vi "XY Galvo.vi"(0 "Exposure /ms":dbl=10.0 format="%0.2p", 1 "FOV max / V":dbl=10.0 format="%0.2p", 2 "Samples per ms":dbl=10.0 format="%0.2p", 3 "Relax /ms":dbl=10.0 format="%0.2p", 4 "FOV min/ V":dbl=10.0 format="%0.2p") -> (5 "XY Galvo":dbl[](graph))   [LabVIEW 2015]
uses:
  GlobalVariables.vi
  <vilib>/Analysis/NI_AALBase.lvlib
panel:
  out "XY Galvo 2":dbl[](graph)
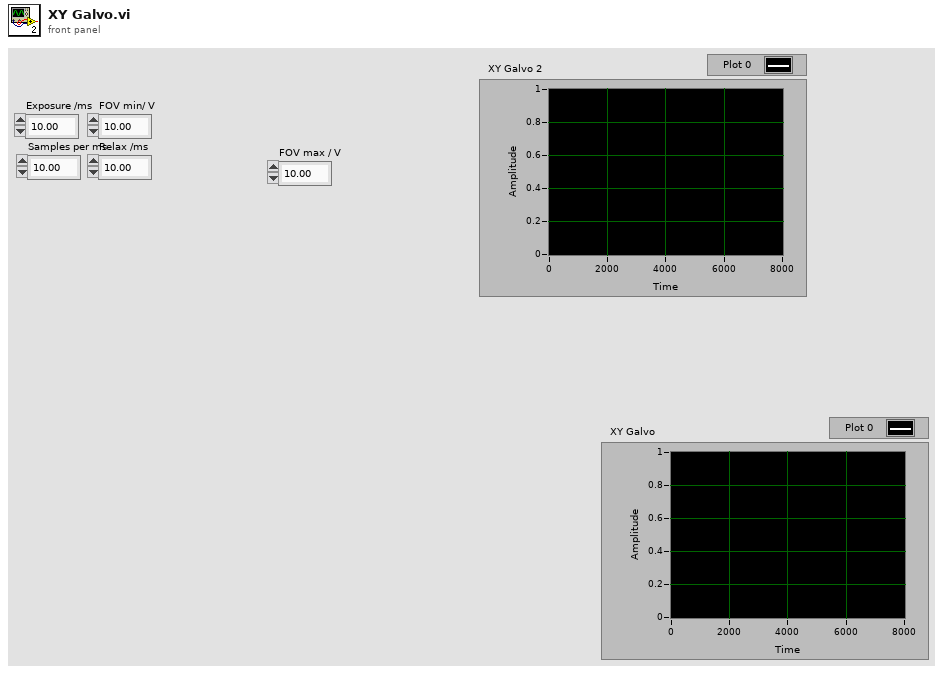
[diagram p1: front panel]
types:
  T1 = cluster{"Top Left":dbl[], "Top Right":dbl[], "Bottom Left":dbl[], "Bottom Right":dbl[]}
  T2 = typedef "NI_Matrix.lvlib/RealMatrix.ctl" = dbl[][]
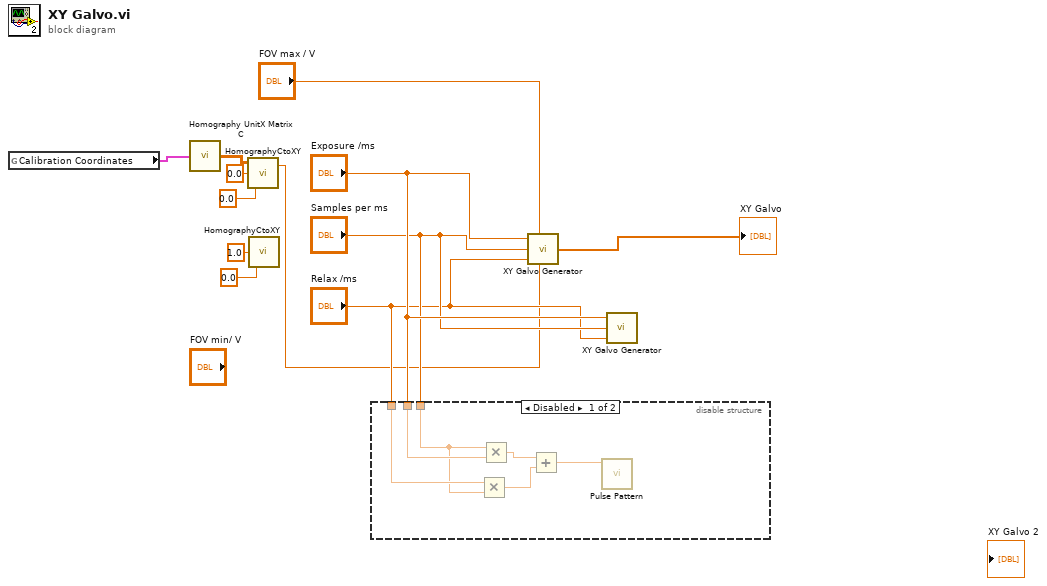
[diagram p0: block diagram]
diagram:
  n1 = global read "GlobalVariables.vi" "Calibration Coordinates"() -> (w7:T1)
  n2 = call "Homography UnitX Matrix C.vi"("input cluster"=w7) -> ("C"=w6:T2)
  n3 = call "HomographyCtoXY.vi"("Y"=0.0, "X"=0.0, "C"=w6) -> ("X"=w1:dbl)  [unwired: 1 out]
  n4 = call "HomographyCtoXY.vi"("Y"=0.0, "X"=1.0) -> ()  [unwired: 1 in, 2 out]
  n5 = disable-structure shown="Disabled" {
    disable-tunnel: "Exposure /ms" -> [w18 _]
    disable-tunnel: "Relax /ms" -> [w17 _]
    disable-tunnel: "Samples per ms" -> [w16 _]
    frame Disabled {
      n6 = Multiply(x=w17, y=w16) -> (x*y=w15:dbl)
      n7 = Multiply(x=w16, y=w18) -> (x*y=w14:dbl)
      n8 = Add(x=w14, y=w15) -> (x+y=w13:dbl)
      n9 = call <vilib>:"Pulse Pattern.vi"("samples"=w13) -> ()  [unwired: 3 in, 2 out]
    }
    frame Enabled {
    }
  }
  n10 = call "XY Galvo Generator.vi"("Exposure /ms"="Exposure /ms", "FOV max / V"="FOV max / V", "Samples per ms"="Samples per ms", "Relax /ms"="Relax /ms", "FOV min/ V"=w1) -> ("Signal"=→"XY Galvo":dbl[])
  n11 = call "XY Galvo Generator.vi"("Exposure /ms"="Exposure /ms", "Samples per ms"="Samples per ms", "Relax /ms"="Relax /ms") -> ()  [unwired: 2 in, 1 out]
